vi "Create Temp VI for Refs.vi"(10 "Block Library":path, 11 "App":refnum<vi>) -> (0 "error out":errorcluster, 3 "VI Name":string)   [LabVIEW 2022 SP3, in "FlexBlocks Support.lvlib"]
uses:
  FlexBlocks Support.lvlib
  <vilib>/Utility/miscctls.llb/LVPointTypeDef.ctl
panel:
  out "VI Refnum":refnum<vi>
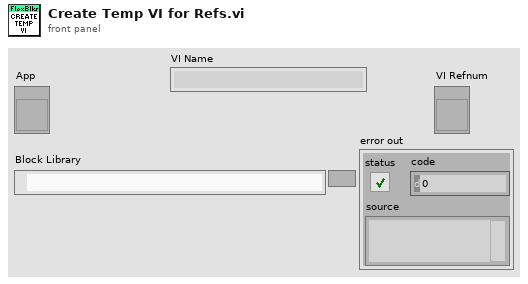
[diagram p1: front panel]
types:
  T1 = enum32{"Invalid", "Standard", "Closed", "Hidden", "Minimized", "Maximized"}
  T2 = typedef "LVPointTypeDef.ctl" = cluster{"Horizontal":i16, "Vertical":i16}
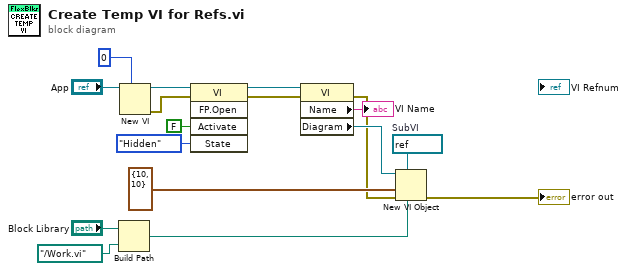
[diagram p0: block diagram]
diagram:
  w8 = refnum<vi> refnum  # SubVI
  n1 = Build Path(base path="Block Library", name or relative path=path "../Work.vi") -> (appended path=w13:path)
  n2 = New VI(7:u32 0 ("options"), 11:"App") -> (0:w2:errorcluster, 3:w7:refnum<vi>)  [unwired: 5 in]
  n3 = invoke class="VI" method="FP.Open"(reference=w7, error in=w2, "Activate"=FALSE ("Activate?"), "State"=T1."Hidden") -> (reference out=w6:refnum<vi>, error out=w5:errorcluster)  [unwired: 1 in, 3 out]
  n4 = property class="VI"(reference=w6, error in=w5) -> (error out=w10:errorcluster, "Name"=→"VI Name":string, "Diagram"=w11:refnum<vi>)  [unwired: 1 out]
  n5 = New VI Object(vi object class=w8, owner refnum=w11, position/next to=T2 {"Horizontal"=10, "Vertical"=10} ("location"), 6:w13, 8:w10) -> (0:→"error out":errorcluster)  [unwired: 3 in, 1 out]
